vi "NavigationKeeper.vi"(6 "intervalo":dbl=0.025 format="%#_13g", 8 "error in (no error)":errorcluster, 10 "Penalty Shoot Out?":bool, 11 "Game in":refnum<class "Game.lvclass">) -> (0 "error out":errorcluster, 3 "Game out":refnum<class "Game.lvclass">)   [LabVIEW 2022 SP3, in "Game.lvclass"]
uses:
  Game.lvclass
  Game.lvclass/Game.ctl
  Parameters_class/Parameters.lvclass/Parameters.ctl
  Read TestMode.vi
  Read Parameters.lvclass.vi
  Parameters_class/Read Project.vi
  Parameters_class/Read MaxAcceleration.vi
  Parameters_class/Read MaxDeceleration.vi
  Parameters_class/Read MaxOutputXY.vi
  Parameters_class/Read MaxOutputAngle.vi
  Parameters_class/Read MaxControlIncrement.vi
  Parameters_class/Read Debug.vi
  Parameters_class/Read PID gains Vel.vi
  Parameters_class/Parameters.lvclass
panel:
  in  "GoTo Navigation":bool
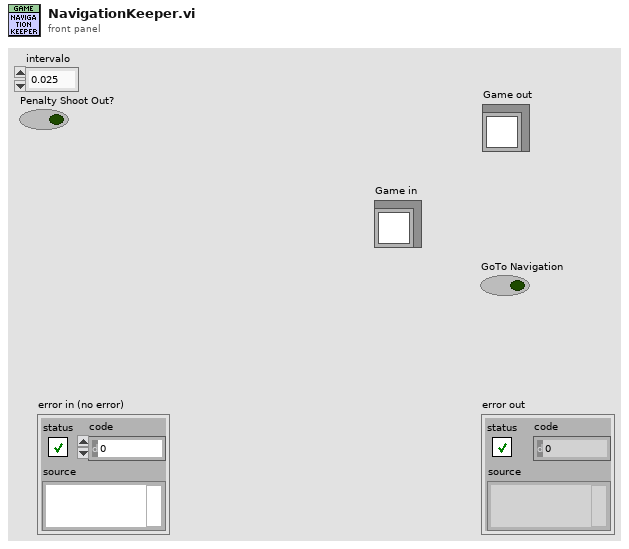
[diagram p1: front panel]
types:
  T1 = typedef "Project.ctl" = enum16{"SSL", "VSS"}
  T2 = cluster{"(Kc)":dbl, "(Ti, min)":dbl, "(Td, min)":dbl}
  T3 = typedef "AI Input.ctl" = cluster{"our_robots":T4[], "enemy_robots":T4[], "balls":T10[], "geometry":T11, "IA Judge":T12, "Received Timestamp":timestamp, "Events":T14}
  T4 = typedef "AI Robot.ctl" = cluster{"id":u32, "function":T5, "x":dbl, "y":dbl, "orientation":dbl, "v_tangent":dbl, "v_normal":dbl, "v_ang":dbl, "kick_x":dbl, "kick_z":dbl, "dribble":bool, "Timestamp":timestamp, "estimatives":cluster{"est_v_tangent":dbl, "est_v_normal":dbl, "est_vx":dbl, "est_vy":dbl, "Pos Robot Est":dbl[]}, "dest_x_kick":dbl, "dest_y_kick":dbl, "Gap Coord":dbl[], "States":T6, "Path ":dbl[][], "Path  Smooth":dbl[][], "Dest":T7, "vx_desired":dbl, "vy_desired":dbl, "slowBehavior":bool, "VSSStates":T9}
  T5 = typedef "Functions Enum.ctl" = enum16{"2nd Striker", "Attacker", "Goalie", "Defender", "Striker", "Goto 0", "Dummy", "Kicker", "ZigZag 0", "ZigZag 1", "ZigZag 2", "ZigZag 3", "ZigZag 4", "ZigZag 5", "ZigZag 6", "ZigZag 7", "ZigZag 8", ""}
  T6 = typedef "AttackerStates.ctl" = enum16{"Pass", "GoToTangent", "BallGetting", "GoToKick", ""}
  T7 = typedef "PathDests.ctl" = T8[]
  T8 = typedef "PathDest.ctl" = cluster{"dest_x":dbl, "dest_y":dbl, "dest_orientation":dbl, "dest_vel":dbl}
  T9 = typedef "VSSAttackerStates.ctl" = enum16{"Pass", "GoToTangent", "BallGetting", "GoToKick", "Rotate anti-clockwise", "Rotate Clockwise", ""}
  T10 = typedef "AI Ball.ctl" = cluster{"x":dbl, "y":dbl, "timestamp":timestamp, "Vel_x":dbl, "Vel_y":dbl, "Pos Bola Est":dbl[], "Valid":bool}
  T11 = typedef "Field Size.ctl" = cluster{"line_width":u32, "field_length":u32, "field_width":u32, "boundary_width":u32, "referee_width":u32, "goal_width":u32, "goal_depth":u32, "goal_wall_width":u32, "center_circle_radius":u32, "defense_radius":u32, "defense_stretch":u32, "free_kick_from_defense_dist":u32, "penalty_spot_from_field_line_dist":u32, "penalty_line_from_spot_dist":u32}
  T12 = typedef "AI Judge.ctl" = cluster{"stage":string, "command":string, "our_goalie_id":dbl, "enemy_goalie_id":dbl, "command enum":T13, "Time":enum16{"Azul", "Amarelo"}}
  T13 = typedef "Command Enum.ctl" = enum16{"Halt", "Stop", "Force Start", "PKA Normal Start", "Prepare Kickoff Ally", "PKE Normal Start", "Prepare Kickoff Enemy", "Prepare Penalty Ally", "PPA Normal Start", "Prepare Penalty Enemy", "PPE Normal Start", "Direct Free Enemy", "Direct Free Ally", "Indirect Free Enemy", "Indirect Free Ally", "Timeout Enemy", "Timeout Ally", "Goal Enemy", "Goal Ally", "Ball Placement Enemy", "Ball Placement Ally", "Normal Half Time", "Extra Time Break", "Extra Half Time", "None", "Post Game"}
  T14 = typedef "Events.ctl" = cluster{"Touch":bool, "Ball out":bool, "id touch":dbl, "Ball out of \nVision":bool, "Ball inside \nGoalie area":bool, "Robot not responding":bool, "Robots responding status":dbl[], "Enemy Ball \nPossession":bool, "Pass State":bool, "id end of pass":dbl, "Kick":bool, "Id ini Possession":dbl, "Ball Possesion":bool, "Id Possesion":dbl, "Direct Kick":bool, "2nd Strk Ativo":bool}
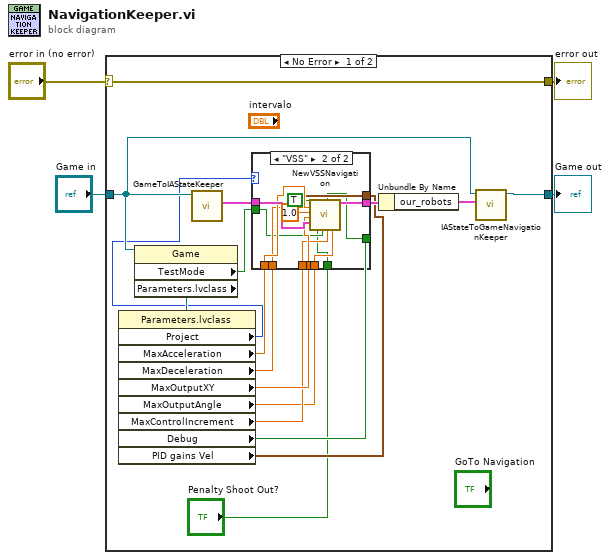
[diagram p0: block diagram]
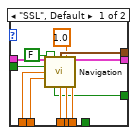
[diagram p2: hidden frame]
diagram:
  n1 = case shown="No Error" "error in (no error)" {
    selector: "error in (no error)" -> [w21 w48]
    tunnel: [w21 w48] -> w3
    tunnel: [w17 w47] -> w1
    tunnel: "Game in" -> [w7 w47]
    frame No Error {
      n2 = property class="Game"(reference=w7) -> ("TestMode"=w8:bool, "Parameters.lvclass"=w16:refnum<class "Parameters.lvclass">)  [unwired: 1 in, 2 out]
      n3 = property class="Parameters.lvclass"(reference=w16) -> ("Project"=w6:T1, "MaxAcceleration"=w15:dbl, "MaxDeceleration"=w14:dbl, "MaxOutputXY"=w13:dbl, "MaxOutputAngle"=w11:dbl, "MaxControlIncrement"=w12:dbl, "Debug"=w10:bool, "PID gains Vel"=w9:T2)  [unwired: 1 in, 2 out]
      n4 = call-dynamic "GameToIAStateKeeper.vi"("Game in"=w7) -> ("IA State out"=w20:T3)  [unwired: 8 in, 2 out]
      n5 = case shown="\"VSS\"" w6 {
        tunnel: w20 -> [w33 w46]
        tunnel: [w32 w45] -> w19
        tunnel: w15 -> [w31 w44]
        tunnel: w14 -> [w30 w43]
        tunnel: w13 -> [w29 w42]
        tunnel: w12 -> [w28 w41]
        tunnel: w11 -> [w27 w40]
        tunnel: w10 -> [w26 w36]
        tunnel: w9 -> [w25 w39]
        tunnel: w8 -> [w24 w38]
        tunnel: "Penalty Shoot Out?" -> [_ w34]
        frame "SSL", Default {
          n6 = call "Navigation.vi"("IA State Output in"=w33, "Penalty Shoot Out?"=FALSE, "PID gains Vel"=w25, "VelNearBall"=1.0, "Test Mode"=w24, "a1"=w31, "a3"=w30, "Debug"=w26, "output inc"=w28, "output xy"=w29, "output angle"=w27) -> ("IA State Output out"=w32:T3)  [unwired: 4 in]
        }
        frame "VSS" {
          n7 = call "NewVSSNavigation.vi"("GoTo Navigation"=TRUE, "a1"=w44, "VelNearBall"=1.0, "output xy"=w42, "IA State Output in"=w46, "a3"=w43, "Penalty Shoot Out?"=w34, "PID gains Vel"=w39, "Test Mode"=w38, "Debug"=w36, "output inc"=w41, "output angle"=w40) -> ("IA State Output out"=w45:T3)  [unwired: 7 in]
        }
      }
      n8 = Unbundle By Name(w19) -> ("our_robots"=w18:T4[])
      n9 = call "IAStateToGameNavigationKeeper.vi"("our_robots"=w18, "Game in"=w7) -> ("Game out"=w17:refnum<class "Game.lvclass">)  [unwired: 8 in, 1 out]
    }
    frame Error {
    }
  }
  "error out" <- w3
  "Game out" <- w1
